vi "get vol info.vi"() -> ()   [LabVIEW 2013]
panel:
  out "volume path":path
  out "free (bytes)":i64
  out "size (bytes)":i64
  in  "path":path
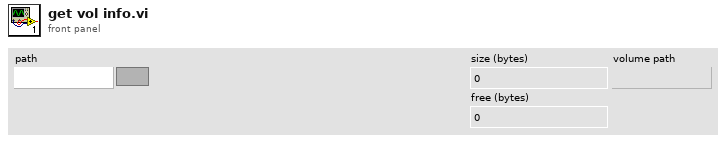
[diagram p1: front panel]
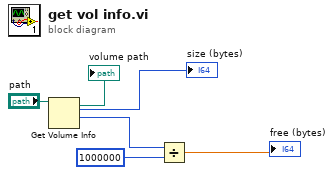
[diagram p0: block diagram]
diagram:
  n1 = Get Volume Info(11:"path") -> (1:w3:i64, 2:→"size (bytes)":i64, 5:→"volume path":path)  [unwired: 1 in, 3 out]
  n2 = Divide(x=w3, y=i64 1000000) -> (x/y=→"free (bytes)":dbl)
